vi "Write FieldDVR.vi"(8 "error in (no error)":errorcluster, 10 "FieldDVR":refnum<data-value>, 11 "Evaluator in":refnum<class "Evaluator.lvclass">) -> (0 "error out":errorcluster, 3 "Evaluator out":refnum<class "Evaluator.lvclass">)   [LabVIEW 2023, in "Evaluator.lvclass"]
uses:
  Evaluator.lvclass
  Field_class/Field.lvclass
  Evaluator.lvclass/Evaluator.ctl
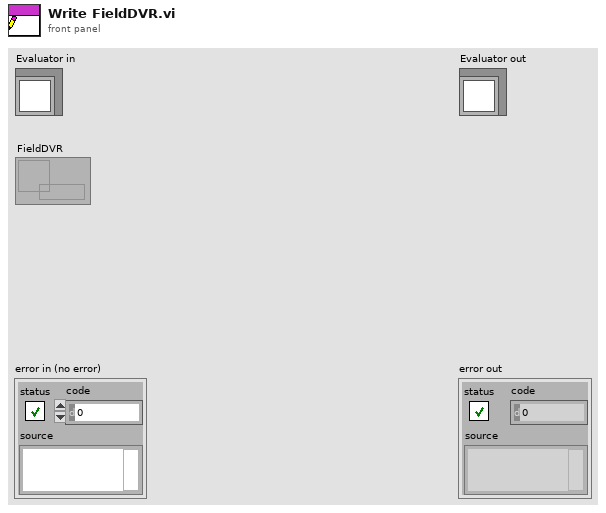
[diagram p1: front panel]
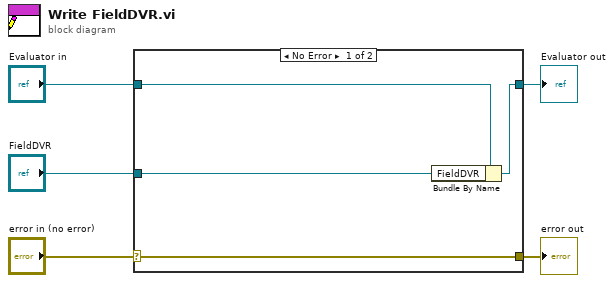
[diagram p0: block diagram]
diagram:
  n1 = case shown="No Error" "error in (no error)" {
    selector: "error in (no error)" -> [w9 w10]
    tunnel: [w9 w10] -> w4
    tunnel: [w7 w11] -> w2
    tunnel: "Evaluator in" -> [w8 w11]
    tunnel: "FieldDVR" -> [w6 _]
    frame No Error {
      n2 = Bundle By Name(cluster=w8, "FieldDVR"=w6) -> (w7:refnum<class "Evaluator.lvclass">)
    }
    frame Error {
    }
  }
  "error out" <- w4
  "Evaluator out" <- w2
